vi "CatchError - log.vi"(8 "error in (no error)":errorcluster) -> (0 "error out":errorcluster)   [LabVIEW 2026, in "Tests.lvlib"]
doc: "Integration test (Caraya): verifies Logger.CatchError catches an incoming error, logs it as exactly one statement at ERROR, and clears the error, with the error dialog suppressed through verbosity (SRS-LMBR-041).\nArranges a manager with the default file off and a Mirror relay capture probe, sets verbosity OFF so the General Error Handler shows no dialog (display is gated independently of the log, SRS-LMBR-042), passes a manufactured error (status TRUE, code 42, source \"T-054 injected\") through CatchError, then asserts the captured statement's level, message, and sourceTag, that CatchError's error out came back cleared, and that no second statement was logged.\nTests.lvlib, friend of Lumberjack.lvlib; runs serially on the shared error wire, cleared at entry for isolation.\n\nImplements LMBR-T-054 -> SRS-041. Assert-level IDs: Test-ID-Assert-Checklist.md."
uses:
  Tests.lvlib
  src/TypeDefs/Severity.ctl
  <vilib>/addons/_JKI Toolkits/Caraya/classes/Assert/Assert Equal Value_Variant.vi
  <vilib>/addons/_JKI Toolkits/Caraya/classes/Assert/Assert False.vi
  <vilib>/addons/_JKI Toolkits/Caraya/classes/Assert/Assert True.vi
  <vilib>/addons/_JKI Toolkits/Caraya/classes/Test/Test.lvclass
  src/Lumberjack.lvlib
  <vilib>/addons/_JKI Toolkits/Caraya/classes/Assert/Assert.lvclass
  src/Public/Logger.lvclass/Logger.lvclass
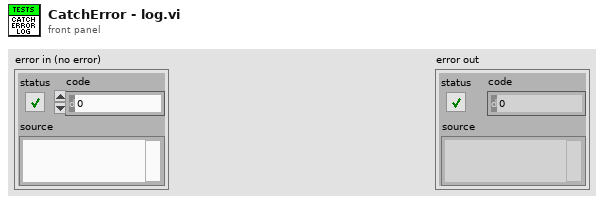
[diagram p1: front panel]
types:
  T1 = typedef "Lumberjack.lvlib/Severity.ctl" = enum16{"OFF", "FATAL", "ERROR", "WARN", "INFO", "DEBUG", "TRACE", "ALL"}
  T2 = typedef "Lumberjack.lvlib/Statement.ctl" = cluster{"timestamp":timestamp, "level":T1, "sourceTag":string, "originVI":string, "message":string}
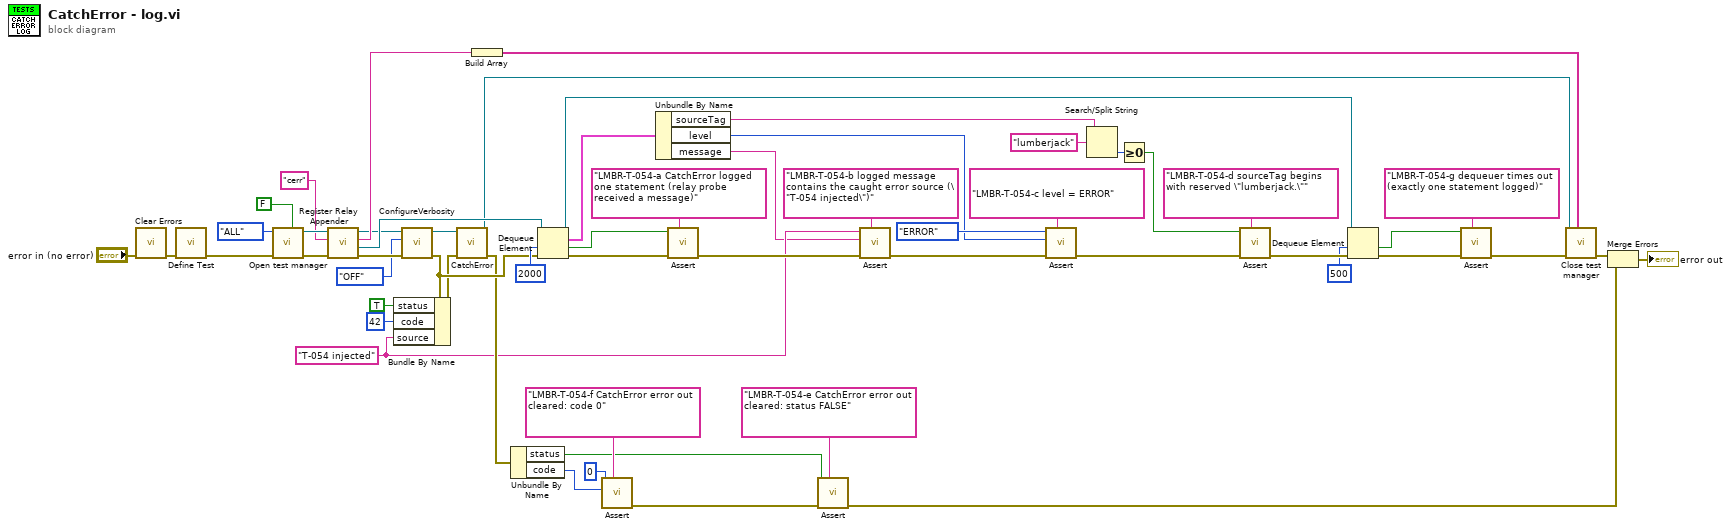
[diagram p0: block diagram]
diagram:
  w15 = "T-054 injected" ("source")
  n1 = call <vilib>:"Clear Errors.vi"("error in (no error)"="error in (no error)") -> ("error out"=w44:errorcluster)  [unwired: 5 in, 1 out]
  n2 = call <vilib>:"Define Test.vi"("error in (no error)"=w44) -> ("error out"=w56:errorcluster)  [unwired: 9 in, 1 out]
  n3 = call "Open test manager.vi"("enableDefaultFile"=FALSE, "error in (no error)"=w56, "globalThreshold"=Severity."ALL") -> ("error out"=w51:errorcluster, "Logger out"=w52:refnum<class "Logger.lvclass">)  [unwired: 7 in]
  n4 = call "Register Relay Appender.vi"("error in (no error)"=w51, "id in"="cerr", "Logger in"=w52) -> ("error out"=w40:errorcluster, "relayQueue"=w50:refnum<queue>, "id out"=w42:string, "Logger out"=w41:refnum<class "Logger.lvclass">)  [unwired: 5 in]
  n5 = call "ConfigureVerbosity.vi"("error in (no error)"=w40, "Verbosity"=Severity."OFF", "Logger in"=w41) -> ("error out"=w38:errorcluster, "Logger out"=w35:refnum<class "Logger.lvclass">)  [unwired: 7 in]
  n6 = Bundle By Name(cluster=w38, "status"=TRUE, "code"=42, "source"=w15) -> (w33:errorcluster)
  n7 = call "CatchError.vi"("error in (no error)"=w33, "Logger in"=w35) -> ("error out"=w32:errorcluster, "Logger out"=w34:refnum<class "Logger.lvclass">)  [unwired: 8 in]
  n8 = Build Array(w42) -> (w49:string[])
  n9 = Unbundle By Name(w32) -> ("status"=w28:bool, "code"=w27:i32)
  n10 = Dequeue Element(queue=w50, timeout in ms (-1)=2000, error in (no error)=w38) -> (queue out=w6:refnum<queue>, element=w53:T2, timed out?=w23:bool, error out=w24:errorcluster)
  n11 = call-poly <vilib>:"Assert.vi"("Label"="LMBR-T-054-f CatchError error out cleared: code 0", "Actual"=w27, "Expected"=0 ("timeout in ms (-1)")) -> ("error out"=w29:errorcluster)  [unwired: 7 in, 1 out]
  n12 = Unbundle By Name(w53) -> ("sourceTag"=w13:string, "level"=w19:T1, "message"=w14:string)
  n13 = call-poly <vilib>:"Assert.vi"("Label"="LMBR-T-054-a CatchError logged one statement (relay probe received a message)", "error in (no error)"=w24, "False?"=w23) -> ("error out"=w17:errorcluster)  [unwired: 7 in, 1 out]
  n14 = call-poly <vilib>:"Assert.vi"("Label"="LMBR-T-054-e CatchError error out cleared: status FALSE", "error in (no error)"=w29, "False?"=w28) -> ("error out"=w3:errorcluster)  [unwired: 7 in, 1 out]
  n15 = call-poly <vilib>:"Assert.vi"("Label"="LMBR-T-054-b logged message contains the caught error source (\"T-054 injected\")", "error in (no error)"=w17, "Actual"=w14, "Expected"=w15) -> ("error out"=w16:errorcluster)  [unwired: 6 in, 1 out]
  n16 = call-poly <vilib>:"Assert.vi"("Label"="LMBR-T-054-c level = ERROR", "error in (no error)"=w16, "Actual"=w19, "Expected"=Severity."ERROR" ("Verbosity")) -> ("error out"=w21:errorcluster)  [unwired: 6 in, 1 out]
  n17 = Search/Split String(string=w13, search string/char (-)="lumberjack") -> (offset of match=w11:i32)  [unwired: 1 in, 2 out]
  n18 = Greater Or Equal To 0?(x=w11) -> (x >= 0?=w10:bool)
  n19 = call-poly <vilib>:"Assert.vi"("Label"="LMBR-T-054-d sourceTag begins with reserved \"lumberjack.\"", "error in (no error)"=w21, "True?"=w10) -> ("error out"=w8:errorcluster)  [unwired: 7 in, 1 out]
  n20 = Dequeue Element(queue=w6, timeout in ms (-1)=500, error in (no error)=w8) -> (timed out?=w4:bool, error out=w7:errorcluster)  [unwired: 2 out]
  n21 = call-poly <vilib>:"Assert.vi"("Label"="LMBR-T-054-g dequeuer times out (exactly one statement logged)", "error in (no error)"=w7, "True?"=w4) -> ("error out"=w9:errorcluster)  [unwired: 7 in, 1 out]
  n22 = call "Close test manager.vi"("queueIDList"=w49, "error in (no error)"=w9, "Logger in"=w34) -> ("error out"=w2:errorcluster)  [unwired: 6 in]
  n23 = Merge Errors(w2, w3) -> (→"error out":errorcluster)
